vi "_WriteTopData_TDMS_Control.vi"(8 "error in (no error)":errorcluster, 10 "Top Data in":T1={"Status"={"id_sensor"=0, "Ind."=FALSE, "sample time"=0, "rov_states"=enum."INIT", "acquisition_time"=timestamp(0 s since 1904-01-01), "modo_ctrl"=enum."Manual"}, "DAQ"={"id_daq"=0, "id_sensor"=0, "gps_"={"lat"=0.0, "lon"=0.0, "alt"=0.0}, "usbl_"={"x"=0.0, "y"=0.0, "z"=0.0}, "vess_ahrs_"={"pitch"=0.0, "roll"=0.0, "yaw"=0.0}, "acquisition_time"=timestamp(0 s since 1904-01-01)}, "User Data"={"id_sensor"=0, "id_daq"=0, "ci_habilitada"=FALSE, "acquisition_time"=timestamp(0 s since 1904-01-01), "CI Data"={"joy_1x"=0.0, "joy_1y"=0.0, "joy_1z"=0.0, "joy_1thumb"=0.0, "joy_1botIzq"=0, "joy_1botder"=0, "joy_1gatillo"=0, "modo_1bot"=0, "modo_2bot"=0, "modo_3bot"=0, "modo_4bot"=0, "pot"=0.0, "enc"=0.0, "joy_2x"=0.0, "joy_2y"=0.0, "joy_2z"=0.0, "joy_2bot"=0, "botella_1bot"=0, "botella_2bot"=0, "botella_3bot"=0, "botella_4bot"=0, "corer_1bot"=0, "corer_2bot"=0, "a_in"=0.0, "dio1"=0, "dio2"=0, "dio3"=0, "ci_acc_x"=0.0, "ci_acc_y"=0.0, "ci_acc_z"=0.0}, "Surface Data"={"modo_1ind"=0, "modo_2ind"=0, "modo_3ind"=0, "modo_4ind"=0, "botella_1ind"=0, "botella_2ind"=0, "botella_3ind"=0, "botella_4ind"=0, "corer_1ind"=0, "corer_2ind"=0, "lars_vel"=0.0, "lars_fwd"=0, "lars_rev"=0}}, "Virtual CI"={"id_sensor"=0, "id_daq"=0, "bus_260v"=FALSE, "m_6"=FALSE, "m_5"=FALSE, "m_2"=FALSE, "m_1"=FALSE, "m_4"=FALSE, "m_3"=FALSE, "luz_1"=FALSE, "luz_2"=FALSE, "luz_3"=FALSE, "pot_m1"=0.0, "pot_m2"=0.0, "pot_m3"=0.0, "pot_m4"=0.0, "pot_m5"=0.0, "pot_m6"=0.0, "pot_l1"=0.0, "pot_l2"=0.0, "pot_l3"=0.0, "pot_gen"=0.0, "fuente_muestras"=FALSE, "bot_1"=FALSE, "bot_2"=FALSE, "bot_3"=FALSE, "bot_4"=FALSE, "corer_1"=FALSE, "corer_2"=FALSE, "pot_c1"=0.0, "pot_c2"=0.0, "virtual_ci"=FALSE, "acquisition_time"=timestamp(0 s since 1904-01-01)}, "Control"={"depth_PID"={"Kp"=0.0, "Ti"=0.03, "Td"=0.001}, "heading_PID"={"Kp"=0.05, "Ti"=0.03, "Td"=0.001}, "altitude_PID"={"Kp"=0.05, "Ti"=0.03, "Td"=0.001}, "depth_sp"=0.0, "heading_sp"=0.0, "altitude_sp"=0.0, "m_PID_en"=FALSE, "PID_reset"=FALSE, "acquisition_time"=timestamp(0 s since 1904-01-01), "motor_PID"={"Kp"=0.05, "Ti"=0.03, "Td"=0.001}, "m1_lo"=0.0, "m1_hi"=0.0, "m1_en"=TRUE, "m2_lo"=0.0, "m2_hi"=0.0, "m2_en"=TRUE, "m3_lo"=0.0, "m3_hi"=0.0, "m3_en"=TRUE, "m4_lo"=0.0, "m4_hi"=5.0, "m4_en"=TRUE, "m5_lo"=-5.0, "m5_hi"=5.0, "m5_en"=TRUE, "m6_lo"=-5.0, "m6_hi"=5.0, "m6_en"=TRUE, "modo_ctrl"=enum."Manual"}} {"Virtual CI"."pot_c2" step=0.1; "Virtual CI"."pot_c1" step=0.01; "Virtual CI"."pot_gen" step=1.0; "Virtual CI"."pot_l3" step=0.01; "Virtual CI"."pot_l2" step=0.01; "Virtual CI"."pot_l1" step=0.01; "Virtual CI"."pot_m6" step=0.01; "Virtual CI"."pot_m5" step=0.01; "Virtual CI"."pot_m4" step=0.01; "Virtual CI"."pot_m3" step=0.01; "Virtual CI"."pot_m2" step=0.01; "Virtual CI"."pot_m1" step=0.01; "DAQ"."vess_ahrs_"."yaw" format="%.2g"; "DAQ"."vess_ahrs_"."roll" format="%.2g"; "DAQ"."vess_ahrs_"."pitch" format="%.2g"; "DAQ"."usbl_"."z" format="%.7g"; "DAQ"."usbl_"."y" format="%.7g"; "DAQ"."usbl_"."x" format="%.7g"; "DAQ"."gps_"."alt" format="%.7g"; "DAQ"."gps_"."lon" format="%.7g"; "DAQ"."gps_"."lat" format="%.7g"}, 11 "Refnum in":refnum<k34>) -> (0 "error out":errorcluster, 3 "Refnum out":refnum<k34>)   [LabVIEW 2018]
uses:
  TypeDefsTopside/Top Data.ctl
  Shared/Type Defs/ROV States.ctl
  TypeDefsSubsea/Modos Control.ctl
  TypeDefsTopside/DAQ Top Data.ctl
  TypeDefsTopside/User Data.ctl
  TypeDefsTopside/CI Data.ctl
  TypeDefsTopside/Surface Input Data.ctl
  TypeDefsTopside/Virtual User Interface Data.ctl
  TypeDefsTopside/Top Control.ctl
  TypeDefsSubsea/Type Defs Subsea.lvlib
  TypeDefsTopside/Type Defs Topside.lvlib
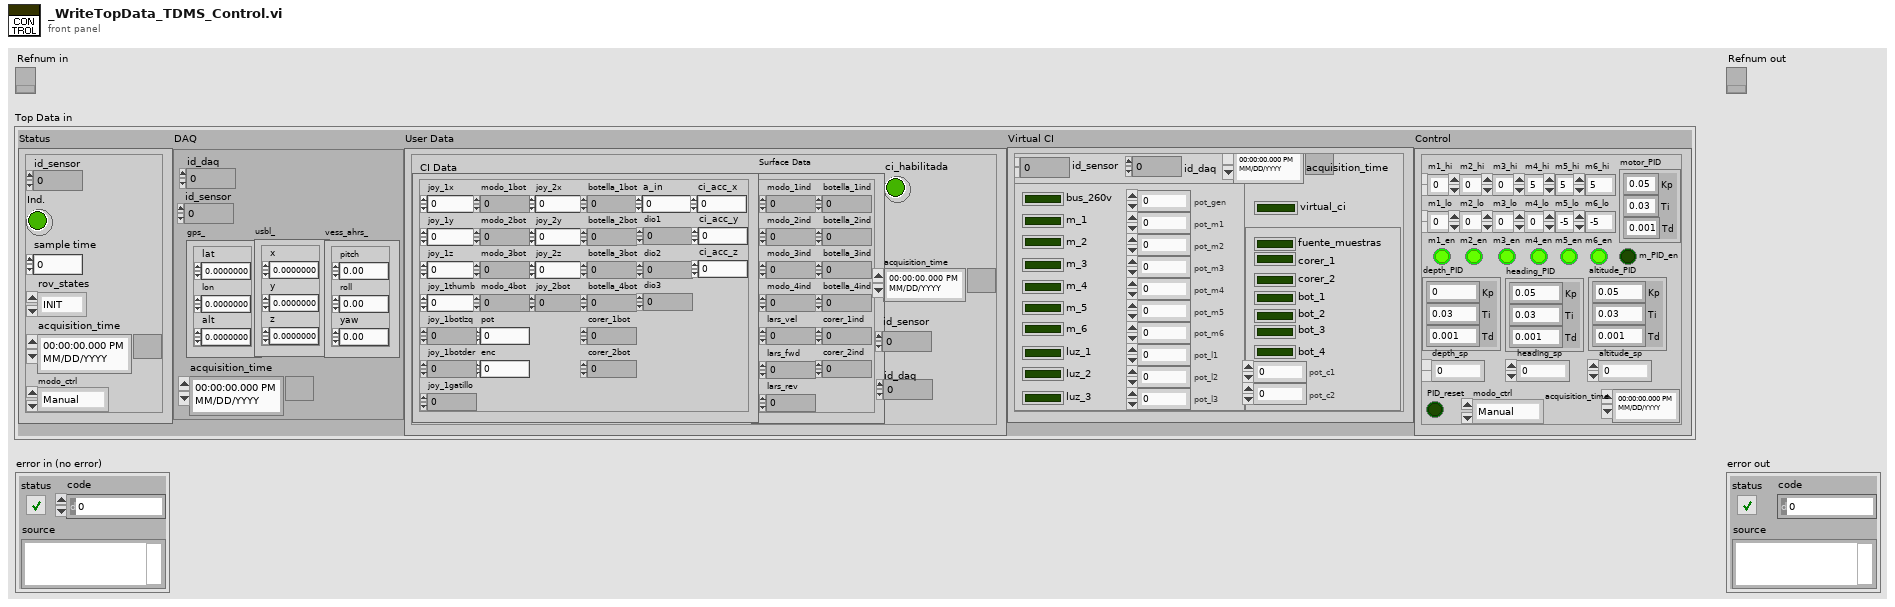
[diagram p1: front panel]
types:
  T1 = typedef "Type Defs Topside.lvlib/Top Data.ctl" = cluster{"Status":cluster{"id_sensor":u32, "Ind.":bool, "sample time":u32, "rov_states":T2, "acquisition_time":timestamp, "modo_ctrl":T3}, "DAQ":T4, "User Data":T5, "Virtual CI":T8, "Control":T9}
  T2 = typedef "Type Defs Subsea.lvlib/ROV States.ctl" = enum16{"INIT", "IDLE", "TEST", "RUN", "EMERGENCY", "EXIT"}
  T3 = typedef "Type Defs Subsea.lvlib/Modos Control.ctl" = enum16{"Manual", "Profundidad", "Altitud", "Rumbo", "P+R"}
  T4 = typedef "Type Defs Topside.lvlib/DAQ Top Data.ctl" = cluster{"id_daq":u32, "id_sensor":u32, "gps_":cluster{"lat":dbl, "lon":dbl, "alt":dbl}, "usbl_":cluster{"x":dbl, "y":dbl, "z":dbl}, "vess_ahrs_":cluster{"pitch":dbl, "roll":dbl, "yaw":dbl}, "acquisition_time":timestamp}
  T5 = typedef "Type Defs Topside.lvlib/User Data.ctl" = cluster{"id_sensor":u32, "id_daq":u64, "ci_habilitada":bool, "acquisition_time":timestamp, "CI Data":T6, "Surface Data":T7}
  T6 = typedef "Type Defs Topside.lvlib/CI Data.ctl" = cluster{"joy_1x":dbl, "joy_1y":dbl, "joy_1z":dbl, "joy_1thumb":dbl, "joy_1botIzq":u8, "joy_1botder":u8, "joy_1gatillo":u8, "modo_1bot":u8, "modo_2bot":u8, "modo_3bot":u8, "modo_4bot":u8, "pot":dbl, "enc":dbl, "joy_2x":dbl, "joy_2y":dbl, "joy_2z":dbl, "joy_2bot":u8, "botella_1bot":u8, "botella_2bot":u8, "botella_3bot":u8, "botella_4bot":u8, "corer_1bot":u8, "corer_2bot":u8, "a_in":dbl, "dio1":u8, "dio2":u8, "dio3":u8, "ci_acc_x":dbl, "ci_acc_y":dbl, "ci_acc_z":dbl}
  T7 = typedef "Type Defs Topside.lvlib/Surface Input Data.ctl" = cluster{"modo_1ind":u8, "modo_2ind":u8, "modo_3ind":u8, "modo_4ind":u8, "botella_1ind":u8, "botella_2ind":u8, "botella_3ind":u8, "botella_4ind":u8, "corer_1ind":u8, "corer_2ind":u8, "lars_vel":dbl, "lars_fwd":u8, "lars_rev":u8}
  T8 = typedef "Type Defs Topside.lvlib/Virtual User Interface Data.ctl" = cluster{"id_sensor":u32, "id_daq":u64, "bus_260v":bool, "m_6":bool, "m_5":bool, "m_2":bool, "m_1":bool, "m_4":bool, "m_3":bool, "luz_1":bool, "luz_2":bool, "luz_3":bool, "pot_m1":dbl, "pot_m2":dbl, "pot_m3":dbl, "pot_m4":dbl, "pot_m5":dbl, "pot_m6":dbl, "pot_l1":dbl, "pot_l2":dbl, "pot_l3":dbl, "pot_gen":dbl, "fuente_muestras":bool, "bot_1":bool, "bot_2":bool, "bot_3":bool, "bot_4":bool, "corer_1":bool, "corer_2":bool, "pot_c1":dbl, "pot_c2":dbl, "virtual_ci":bool, "acquisition_time":timestamp}
  T9 = typedef "Type Defs Topside.lvlib/Top Control.ctl" = cluster{"depth_PID":cluster{"Kp":dbl, "Ti":dbl, "Td":dbl}, "heading_PID":cluster{"Kp":dbl, "Ti":dbl, "Td":dbl}, "altitude_PID":cluster{"Kp":dbl, "Ti":dbl, "Td":dbl}, "depth_sp":dbl, "heading_sp":dbl, "altitude_sp":dbl, "m_PID_en":bool, "PID_reset":bool, "acquisition_time":timestamp, "motor_PID":cluster{"Kp":dbl, "Ti":dbl, "Td":dbl}, "m1_lo":dbl, "m1_hi":dbl, "m1_en":bool, "m2_lo":dbl, "m2_hi":dbl, "m2_en":bool, "m3_lo":dbl, "m3_hi":dbl, "m3_en":bool, "m4_lo":dbl, "m4_hi":dbl, "m4_en":bool, "m5_lo":dbl, "m5_hi":dbl, "m5_en":bool, "m6_lo":dbl, "m6_hi":dbl, "m6_en":bool, "modo_ctrl":T3}
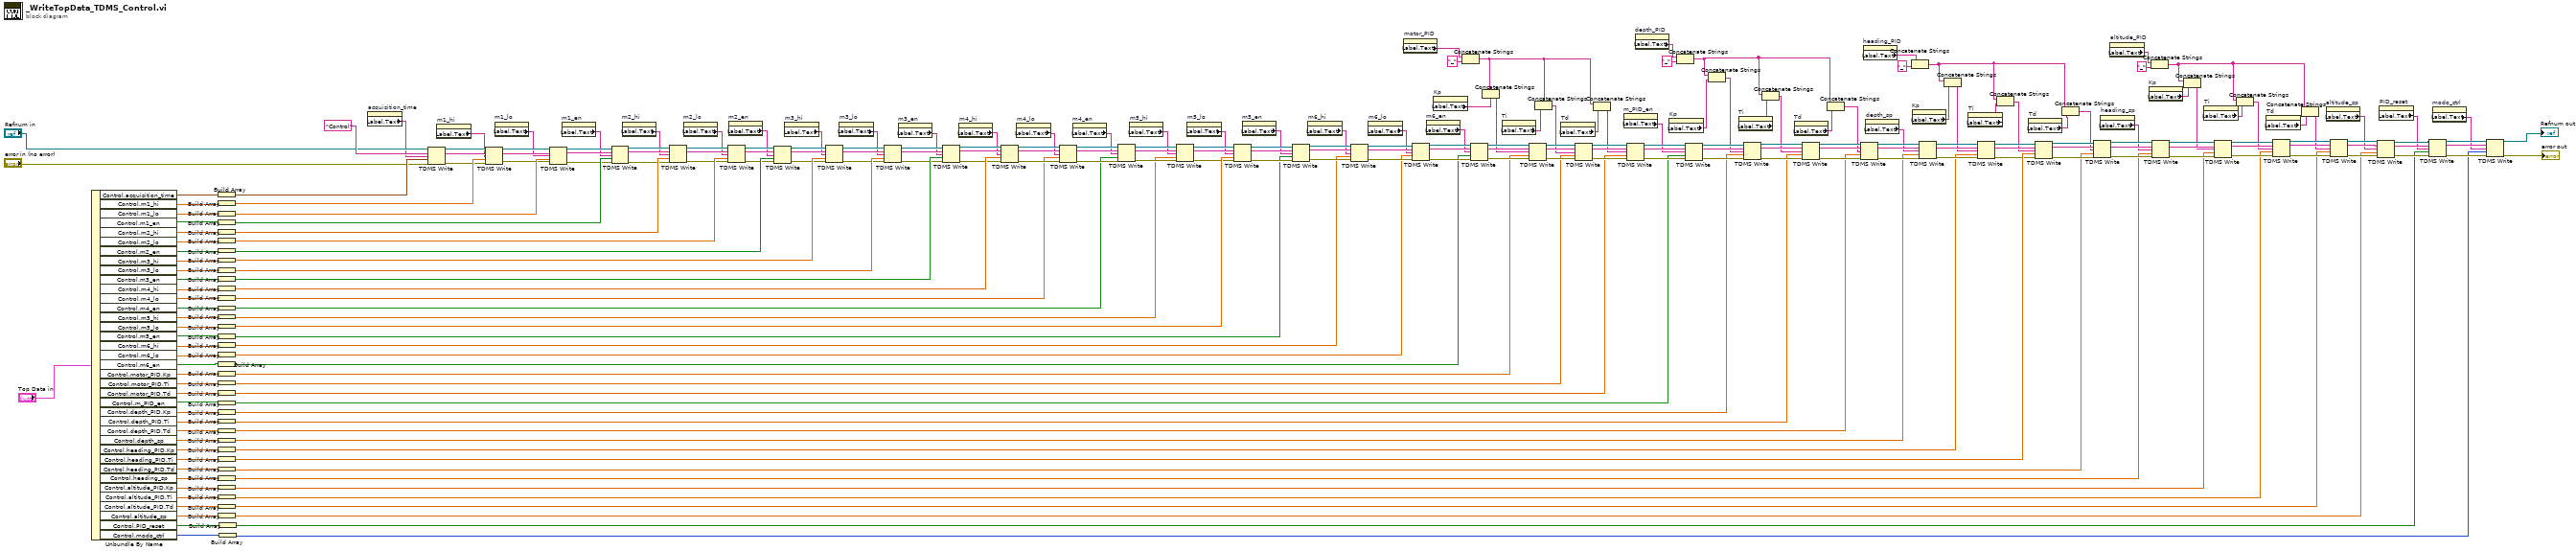
[diagram p0: block diagram]
diagram:
  n1 = Unbundle By Name("Top Data in") -> ("Control.acquisition_time"=w238:timestamp, "Control.m1_hi"=w96:dbl, "Control.m1_lo"=w95:dbl, "Control.m1_en"=w94:bool, "Control.m2_hi"=w93:dbl, "Control.m2_lo"=w92:dbl, "Control.m2_en"=w91:bool, "Control.m3_hi"=w90:dbl, "Control.m3_lo"=w89:dbl, "Control.m3_en"=w88:bool, "Control.m4_hi"=w87:dbl, "Control.m4_lo"=w86:dbl, "Control.m4_en"=w85:bool, "Control.m5_hi"=w84:dbl, "Control.m5_lo"=w83:dbl, "Control.m5_en"=w82:bool, "Control.m6_hi"=w81:dbl, "Control.m6_lo"=w80:dbl, "Control.m6_en"=w79:bool, "Control.motor_PID.Kp"=w78:dbl, "Control.motor_PID.Ti"=w77:dbl, "Control.motor_PID.Td"=w76:dbl, "Control.m_PID_en"=w75:bool, "Control.depth_PID.Kp"=w74:dbl, "Control.depth_PID.Ti"=w73:dbl, "Control.depth_PID.Td"=w72:dbl, "Control.depth_sp"=w71:dbl, "Control.heading_PID.Kp"=w70:dbl, "Control.heading_PID.Ti"=w69:dbl, "Control.heading_PID.Td"=w68:dbl, "Control.heading_sp"=w67:dbl, "Control.altitude_PID.Kp"=w66:dbl, "Control.altitude_PID.Ti"=w65:dbl, "Control.altitude_PID.Td"=w64:dbl, "Control.altitude_sp"=w63:dbl, "Control.PID_reset"=w62:bool, "Control.modo_ctrl"=w61:T3)
  n2 = Build Array(w238) -> (w239:timestamp[])
  n3 = Build Array(w96) -> (w240:dbl[])
  n4 = Build Array(w95) -> (w241:dbl[])
  n5 = Build Array(w94) -> (w242:bool[])
  n6 = Build Array(w93) -> (w243:dbl[])
  n7 = Build Array(w92) -> (w244:dbl[])
  n8 = Build Array(w91) -> (w245:bool[])
  n9 = Build Array(w90) -> (w246:dbl[])
  n10 = Build Array(w89) -> (w247:dbl[])
  n11 = Build Array(w88) -> (w248:bool[])
  n12 = Build Array(w87) -> (w249:dbl[])
  n13 = Build Array(w86) -> (w204:dbl[])
  n14 = Build Array(w85) -> (w203:bool[])
  n15 = Build Array(w84) -> (w202:dbl[])
  n16 = Build Array(w83) -> (w131:dbl[])
  n17 = Build Array(w82) -> (w130:bool[])
  n18 = Build Array(w81) -> (w129:dbl[])
  n19 = Build Array(w80) -> (w128:dbl[])
  n20 = Build Array(w79) -> (w127:bool[])
  n21 = Build Array(w78) -> (w126:dbl[])
  n22 = Build Array(w77) -> (w125:dbl[])
  n23 = Build Array(w76) -> (w124:dbl[])
  n24 = Build Array(w75) -> (w123:bool[])
  n25 = Build Array(w74) -> (w122:dbl[])
  n26 = Build Array(w73) -> (w121:dbl[])
  n27 = Build Array(w72) -> (w120:dbl[])
  n28 = Build Array(w71) -> (w119:dbl[])
  n29 = Build Array(w70) -> (w118:dbl[])
  n30 = Build Array(w69) -> (w117:dbl[])
  n31 = Build Array(w68) -> (w116:dbl[])
  n32 = Build Array(w67) -> (w115:dbl[])
  n33 = Build Array(w66) -> (w114:dbl[])
  n34 = Build Array(w65) -> (w113:dbl[])
  n35 = Build Array(w64) -> (w112:dbl[])
  n36 = Build Array(w63) -> (w111:dbl[])
  n37 = Build Array(w62) -> (w110:bool[])
  n38 = Build Array(w61) -> (w109:T3[])
  n39 = property on="acquisition_time" class="AbsTime (strict)"() -> ("Label.Text"=w97:string)  [unwired: 2 in, 2 out]
  n40 = TDMS Write(0:"Refnum in", 5:"Control" ("group name in (Untitled)"), 7:w97, 9:w239, 11:"error in (no error)") -> (4:w214:refnum<k34>, 6:w213:string, 15:w215:errorcluster)  [unwired: 1 in, 1 out]
  n41 = property on="m1_hi" class="DigNum (strict)"() -> ("Label.Text"=w60:string)  [unwired: 2 in, 2 out]
  n42 = TDMS Write(0:w214, 5:w213, 7:w60, 9:w240, 11:w215) -> (4:w100:refnum<k34>, 6:w99:string, 15:w98:errorcluster)  [unwired: 1 in, 1 out]
  n43 = property on="m1_lo" class="DigNum (strict)"() -> ("Label.Text"=w58:string)  [unwired: 2 in, 2 out]
  n44 = TDMS Write(0:w100, 5:w99, 7:w58, 9:w241, 11:w98) -> (4:w200:refnum<k34>, 6:w199:string, 15:w201:errorcluster)  [unwired: 1 in, 1 out]
  n45 = property on="m1_en" class="Bool (strict)"() -> ("Label.Text"=w57:string)  [unwired: 2 in, 2 out]
  n46 = TDMS Write(0:w200, 5:w199, 7:w57, 9:w242, 11:w201) -> (4:w218:refnum<k34>, 6:w219:string, 15:w217:errorcluster)  [unwired: 1 in, 1 out]
  n47 = property on="m2_hi" class="DigNum (strict)"() -> ("Label.Text"=w56:string)  [unwired: 2 in, 2 out]
  n48 = TDMS Write(0:w218, 5:w219, 7:w56, 9:w243, 11:w217) -> (4:w221:refnum<k34>, 6:w222:string, 15:w220:errorcluster)  [unwired: 1 in, 1 out]
  n49 = property on="m2_lo" class="DigNum (strict)"() -> ("Label.Text"=w55:string)  [unwired: 2 in, 2 out]
  n50 = TDMS Write(0:w221, 5:w222, 7:w55, 9:w244, 11:w220) -> (4:w234:refnum<k34>, 6:w236:string, 15:w235:errorcluster)  [unwired: 1 in, 1 out]
  n51 = property on="m2_en" class="Bool (strict)"() -> ("Label.Text"=w54:string)  [unwired: 2 in, 2 out]
  n52 = TDMS Write(0:w234, 5:w236, 7:w54, 9:w245, 11:w235) -> (4:w232:refnum<k34>, 6:w233:string, 15:w237:errorcluster)  [unwired: 1 in, 1 out]
  n53 = property on="m3_hi" class="DigNum (strict)"() -> ("Label.Text"=w53:string)  [unwired: 2 in, 2 out]
  n54 = TDMS Write(0:w232, 5:w233, 7:w53, 9:w246, 11:w237) -> (4:w230:refnum<k34>, 6:w231:string, 15:w229:errorcluster)  [unwired: 1 in, 1 out]
  n55 = property on="m3_lo" class="DigNum (strict)"() -> ("Label.Text"=w52:string)  [unwired: 2 in, 2 out]
  n56 = TDMS Write(0:w230, 5:w231, 7:w52, 9:w247, 11:w229) -> (4:w224:refnum<k34>, 6:w225:string, 15:w223:errorcluster)  [unwired: 1 in, 1 out]
  n57 = property on="m3_en" class="Bool (strict)"() -> ("Label.Text"=w51:string)  [unwired: 2 in, 2 out]
  n58 = TDMS Write(0:w224, 5:w225, 7:w51, 9:w248, 11:w223) -> (4:w227:refnum<k34>, 6:w228:string, 15:w226:errorcluster)  [unwired: 1 in, 1 out]
  n59 = property on="m4_hi" class="DigNum (strict)"() -> ("Label.Text"=w50:string)  [unwired: 2 in, 2 out]
  n60 = TDMS Write(0:w227, 5:w228, 7:w50, 9:w249, 11:w226) -> (4:w206:refnum<k34>, 6:w198:string, 15:w205:errorcluster)  [unwired: 1 in, 1 out]
  n61 = property on="m4_lo" class="DigNum (strict)"() -> ("Label.Text"=w49:string)  [unwired: 2 in, 2 out]
  n62 = TDMS Write(0:w206, 5:w198, 7:w49, 9:w204, 11:w205) -> (4:w208:refnum<k34>, 6:w209:string, 15:w207:errorcluster)  [unwired: 1 in, 1 out]
  n63 = property on="m4_en" class="Bool (strict)"() -> ("Label.Text"=w48:string)  [unwired: 2 in, 2 out]
  n64 = TDMS Write(0:w208, 5:w209, 7:w48, 9:w203, 11:w207) -> (4:w211:refnum<k34>, 6:w212:string, 15:w210:errorcluster)  [unwired: 1 in, 1 out]
  n65 = property on="m5_hi" class="DigNum (strict)"() -> ("Label.Text"=w47:string)  [unwired: 2 in, 2 out]
  n66 = TDMS Write(0:w211, 5:w212, 7:w47, 9:w202, 11:w210) -> (4:w104:refnum<k34>, 6:w102:string, 15:w103:errorcluster)  [unwired: 1 in, 1 out]
  n67 = property on="m5_lo" class="DigNum (strict)"() -> ("Label.Text"=w46:string)  [unwired: 2 in, 2 out]
  n68 = TDMS Write(0:w104, 5:w102, 7:w46, 9:w131, 11:w103) -> (4:w174:refnum<k34>, 6:w173:string, 15:w175:errorcluster)  [unwired: 1 in, 1 out]
  n69 = property on="m5_en" class="Bool (strict)"() -> ("Label.Text"=w45:string)  [unwired: 2 in, 2 out]
  n70 = TDMS Write(0:w174, 5:w173, 7:w45, 9:w130, 11:w175) -> (4:w171:refnum<k34>, 6:w170:string, 15:w172:errorcluster)  [unwired: 1 in, 1 out]
  n71 = property on="m6_hi" class="DigNum (strict)"() -> ("Label.Text"=w44:string)  [unwired: 2 in, 2 out]
  n72 = TDMS Write(0:w171, 5:w170, 7:w44, 9:w129, 11:w172) -> (4:w160:refnum<k34>, 6:w159:string, 15:w161:errorcluster)  [unwired: 1 in, 1 out]
  n73 = property on="m6_lo" class="DigNum (strict)"() -> ("Label.Text"=w43:string)  [unwired: 2 in, 2 out]
  n74 = property on="motor_PID" class="Clust (strict)"() -> ("Label.Text"=w41:string)  [unwired: 2 in, 2 out]
  n75 = TDMS Write(0:w160, 5:w159, 7:w43, 9:w128, 11:w161) -> (4:w177:refnum<k34>, 6:w178:string, 15:w176:errorcluster)  [unwired: 1 in, 1 out]
  n76 = property on="m6_en" class="Bool (strict)"() -> ("Label.Text"=w42:string)  [unwired: 2 in, 2 out]
  n77 = property on="Kp" class="DigNum (strict)"() -> ("Label.Text"=w40:string)  [unwired: 2 in, 2 out]
  n78 = Concatenate Strings(w41, "_" ("string")) -> (w36:string)
  n79 = TDMS Write(0:w177, 5:w178, 7:w42, 9:w127, 11:w176) -> (4:w180:refnum<k34>, 6:w181:string, 15:w179:errorcluster)  [unwired: 1 in, 1 out]
  n80 = Concatenate Strings(w36, w40) -> (w39:string)
  n81 = property on="Ti" class="DigNum (strict)"() -> ("Label.Text"=w28:string)  [unwired: 2 in, 2 out]
  n82 = TDMS Write(0:w180, 5:w181, 7:w39, 9:w126, 11:w179) -> (4:w193:refnum<k34>, 6:w195:string, 15:w194:errorcluster)  [unwired: 1 in, 1 out]
  n83 = Concatenate Strings(w36, w28) -> (w38:string)
  n84 = property on="Td" class="DigNum (strict)"() -> ("Label.Text"=w29:string)  [unwired: 2 in, 2 out]
  n85 = TDMS Write(0:w193, 5:w195, 7:w38, 9:w125, 11:w194) -> (4:w191:refnum<k34>, 6:w192:string, 15:w196:errorcluster)  [unwired: 1 in, 1 out]
  n86 = Concatenate Strings(w36, w29) -> (w37:string)
  n87 = property on="m_PID_en" class="Bool (strict)"() -> ("Label.Text"=w23:string)  [unwired: 2 in, 2 out]
  n88 = TDMS Write(0:w191, 5:w192, 7:w37, 9:w124, 11:w196) -> (4:w189:refnum<k34>, 6:w190:string, 15:w188:errorcluster)  [unwired: 1 in, 1 out]
  n89 = property on="depth_PID" class="Clust (strict)"() -> ("Label.Text"=w33:string)  [unwired: 2 in, 2 out]
  n90 = property on="Kp" class="DigNum (strict)"() -> ("Label.Text"=w32:string)  [unwired: 2 in, 2 out]
  n91 = Concatenate Strings(w33, "_" ("string")) -> (w34:string)
  n92 = TDMS Write(0:w189, 5:w190, 7:w23, 9:w123, 11:w188) -> (4:w183:refnum<k34>, 6:w184:string, 15:w182:errorcluster)  [unwired: 1 in, 1 out]
  n93 = Concatenate Strings(w34, w32) -> (w21:string)
  n94 = property on="Ti" class="DigNum (strict)"() -> ("Label.Text"=w31:string)  [unwired: 2 in, 2 out]
  n95 = TDMS Write(0:w183, 5:w184, 7:w21, 9:w122, 11:w182) -> (4:w186:refnum<k34>, 6:w187:string, 15:w185:errorcluster)  [unwired: 1 in, 1 out]
  n96 = Concatenate Strings(w34, w31) -> (w22:string)
  n97 = property on="Td" class="DigNum (strict)"() -> ("Label.Text"=w30:string)  [unwired: 2 in, 2 out]
  n98 = TDMS Write(0:w186, 5:w187, 7:w22, 9:w121, 11:w185) -> (4:w163:refnum<k34>, 6:w158:string, 15:w162:errorcluster)  [unwired: 1 in, 1 out]
  n99 = Concatenate Strings(w34, w30) -> (w20:string)
  n100 = TDMS Write(0:w163, 5:w158, 7:w20, 9:w120, 11:w162) -> (4:w165:refnum<k34>, 6:w166:string, 15:w164:errorcluster)  [unwired: 1 in, 1 out]
  n101 = property on="heading_PID" class="Clust (strict)"() -> ("Label.Text"=w17:string)  [unwired: 2 in, 2 out]
  n102 = property on="depth_sp" class="DigNum (strict)"() -> ("Label.Text"=w19:string)  [unwired: 2 in, 2 out]
  n103 = Concatenate Strings(w17, "_" ("string")) -> (w26:string)
  n104 = property on="Kp" class="DigNum (strict)"() -> ("Label.Text"=w18:string)  [unwired: 2 in, 2 out]
  n105 = TDMS Write(0:w165, 5:w166, 7:w19, 9:w119, 11:w164) -> (4:w168:refnum<k34>, 6:w169:string, 15:w167:errorcluster)  [unwired: 1 in, 1 out]
  n106 = Concatenate Strings(w26, w18) -> (w14:string)
  n107 = property on="Ti" class="DigNum (strict)"() -> ("Label.Text"=w16:string)  [unwired: 2 in, 2 out]
  n108 = TDMS Write(0:w168, 5:w169, 7:w14, 9:w118, 11:w167) -> (4:w107:refnum<k34>, 6:w101:string, 15:w108:errorcluster)  [unwired: 1 in, 1 out]
  n109 = Concatenate Strings(w26, w16) -> (w13:string)
  n110 = property on="Td" class="DigNum (strict)"() -> ("Label.Text"=w15:string)  [unwired: 2 in, 2 out]
  n111 = TDMS Write(0:w107, 5:w101, 7:w13, 9:w117, 11:w108) -> (4:w139:refnum<k34>, 6:w138:string, 15:w140:errorcluster)  [unwired: 1 in, 1 out]
  n112 = Concatenate Strings(w26, w15) -> (w12:string)
  n113 = TDMS Write(0:w139, 5:w138, 7:w12, 9:w116, 11:w140) -> (4:w136:refnum<k34>, 6:w135:string, 15:w137:errorcluster)  [unwired: 1 in, 1 out]
  n114 = property on="heading_sp" class="DigNum (strict)"() -> ("Label.Text"=w11:string)  [unwired: 2 in, 2 out]
  n115 = property on="altitude_PID" class="Clust (strict)"() -> ("Label.Text"=w1:string)  [unwired: 2 in, 2 out]
  n116 = property on="Kp" class="DigNum (strict)"() -> ("Label.Text"=w10:string)  [unwired: 2 in, 2 out]
  n117 = Concatenate Strings(w1, "_" ("string")) -> (w24:string)
  n118 = TDMS Write(0:w136, 5:w135, 7:w11, 9:w115, 11:w137) -> (4:w133:refnum<k34>, 6:w132:string, 15:w134:errorcluster)  [unwired: 1 in, 1 out]
  n119 = Concatenate Strings(w24, w10) -> (w7:string)
  n120 = property on="Ti" class="DigNum (strict)"() -> ("Label.Text"=w9:string)  [unwired: 2 in, 2 out]
  n121 = TDMS Write(0:w133, 5:w132, 7:w7, 9:w114, 11:w134) -> (4:w142:refnum<k34>, 6:w143:string, 15:w141:errorcluster)  [unwired: 1 in, 1 out]
  n122 = Concatenate Strings(w24, w9) -> (w6:string)
  n123 = property on="Td" class="DigNum (strict)"() -> ("Label.Text"=w8:string)  [unwired: 2 in, 2 out]
  n124 = TDMS Write(0:w142, 5:w143, 7:w6, 9:w113, 11:w141) -> (4:w145:refnum<k34>, 6:w146:string, 15:w144:errorcluster)  [unwired: 1 in, 1 out]
  n125 = Concatenate Strings(w24, w8) -> (w5:string)
  n126 = property on="altitude_sp" class="DigNum (strict)"() -> ("Label.Text"=w4:string)  [unwired: 2 in, 2 out]
  n127 = TDMS Write(0:w145, 5:w146, 7:w5, 9:w112, 11:w144) -> (4:w154:refnum<k34>, 6:w156:string, 15:w155:errorcluster)  [unwired: 1 in, 1 out]
  n128 = TDMS Write(0:w154, 5:w156, 7:w4, 9:w111, 11:w155) -> (4:w152:refnum<k34>, 6:w153:string, 15:w157:errorcluster)  [unwired: 1 in, 1 out]
  n129 = property on="PID_reset" class="Bool (strict)"() -> ("Label.Text"=w3:string)  [unwired: 2 in, 2 out]
  n130 = TDMS Write(0:w152, 5:w153, 7:w3, 9:w110, 11:w157) -> (4:w150:refnum<k34>, 6:w151:string, 15:w149:errorcluster)  [unwired: 1 in, 1 out]
  n131 = property on="modo_ctrl" class="Enum (strict)"() -> ("Label.Text"=w2:string)  [unwired: 2 in, 2 out]
  n132 = TDMS Write(0:w150, 5:w151, 7:w2, 9:w109, 11:w149) -> (4:→"Refnum out":refnum<k34>, 15:→"error out":errorcluster)  [unwired: 1 in, 2 out]
